vi "Assert Not Error.vi"(7 "Message (\"\")":string, 8 "error in (no error)":errorcluster) -> (0 "error out":errorcluster)   [LabVIEW 2017, in "Transparent Assertions.lvlib" / "Assertions.lvlib"]
doc: "Asserts that <B>error in</B> is no error. Returns an error if the assertion failed. Optionally adds a message to the error message if the assertion failed."
uses:
  Assertions.lvlib
  Constraints/Error/ErrorType.ctl
  Constraints/Error/Error.lvclass
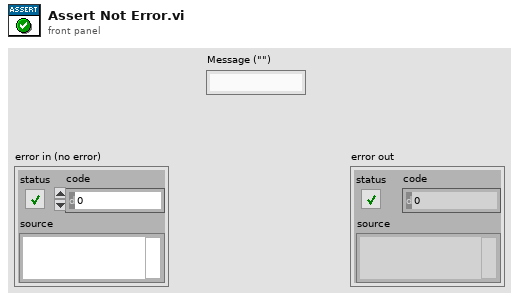
[diagram p1: front panel]
types:
  T1 = typedef "Transparent Assertions.lvlib/Constraints.lvlib/Error.lvclass/ErrorType.ctl" = enum16{"error", "warning", "no error"}
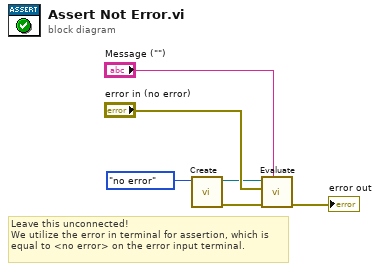
[diagram p0: block diagram]
diagram:
  # "Leave this unconnected!\nWe utilize the error in terminal for assertion, which is\nequal to <no error> on the error input terminal."
  n1 = call "Create.vi"("ErrorType"=ErrorType."no error") -> ("error out"=w2:errorcluster, "Error"=w1:refnum<class "Error.lvclass">)  [unwired: 9 in]
  n2 = call-dynamic "Evaluate.vi"("Message (\"\")"="Message (\"\")", "error in (no error)"=w2, "Actual"="error in (no error)", "Constraint in"=w1) -> ("error out"=→"error out":errorcluster)  [unwired: 6 in, 1 out]
